vi "fitROI.vi"(0 "HGF_IMAQDevice in":refnum<class "HGF_IMAQDevice.lvclass">, 1 "Region of Interest In":i32[](array[numeric]), 2 "Fit Mode":u32(ring) items=["Larger", "Smaller"], 5 "error in (no error)":errorcluster) -> (14 "HGF_IMAQDevice out":refnum<class "HGF_IMAQDevice.lvclass">, 15 "Region of Interest Out":i32[](array[numeric]), 19 "error out":errorcluster)   [LabVIEW 2014, in "HGF_IMAQ.lvlib" / "HGF_IMAQDevice.lvclass"]
doc: "Evaluates the region of interest (ROI) you specify, and returns valid left, top, height, and width values."
uses:
  HGF_IMAQDevice.lvclass
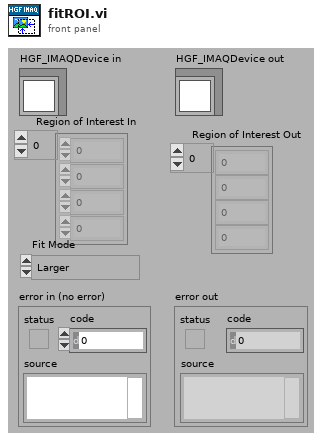
[diagram p1: front panel]
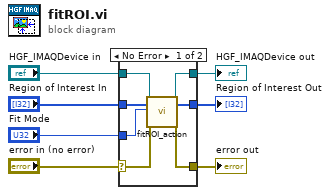
[diagram p0: block diagram]
diagram:
  n1 = case shown="No Error" "error in (no error)" {
    selector: "error in (no error)" -> [w12 w17]
    tunnel: [w11 w17] -> w6
    tunnel: [w13 w16] -> w4
    tunnel: "HGF_IMAQDevice in" -> [w14 w16]
    tunnel: "Region of Interest In" -> [w10 w15]
    tunnel: [w9 w15] -> w2
    tunnel: "Fit Mode" -> [w8 _]
    frame No Error {
      n2 = call-dynamic "fitROI_action.vi"("HGF_IMAQDevice in"=w14, "Region of Interest In"=w10, "Fit Mode"=w8, "error in (no error)"=w12) -> ("HGF_IMAQDevice out"=w13:refnum<class "HGF_IMAQDevice.lvclass">, "Region of Interest Out"=w9:i32[], "error out"=w11:errorcluster)  [unwired: 13 in]
    }
    frame Error {
    }
  }
  "error out" <- w6
  "HGF_IMAQDevice out" <- w4
  "Region of Interest Out" <- w2
